vi "GetPosition.vi"(9 "连接ID":refnum<k5>) -> (0 "y":dbl, 1 "x":dbl, 3 "连接ID 2":refnum<k5>, 4 "c":dbl)   [LabVIEW 2016]
panel:
  out "数据输出":string
  in  "错误输入（无错误）":errorcluster
  out "error out":errorcluster
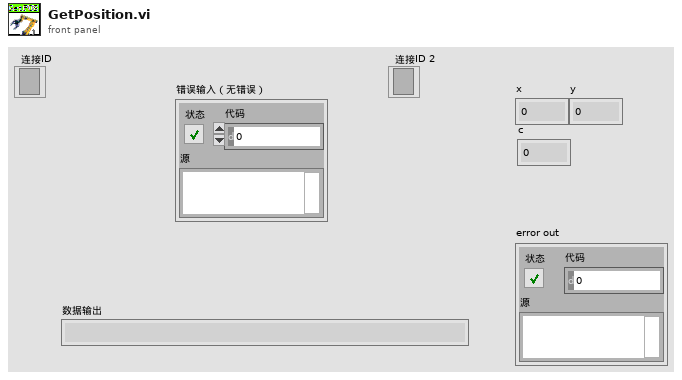
[diagram p1: front panel]
types:
  T1 = enum16{"Standard", "Buffered", "CRLF", "Immediate"}
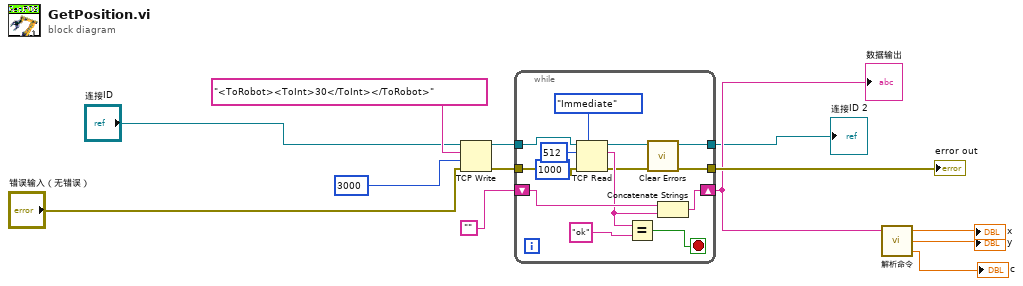
[diagram p0: block diagram]
diagram:
  n1 = TCP Write(connection ID="连接ID", data in="<ToRobot><ToInt>30</ToInt></ToRobot>", error in (no error)="错误输入（无错误）", 9:3000 ("超时毫秒(25000)")) -> (connection ID out=w11:refnum<k5>, error out=w8:errorcluster)  [unwired: 1 out]
  n2 = while {
    shift-right: [w17] -> w7
    shift-left: "" -> [w18]
    tunnel: w11 -> [w25]
    tunnel: [w26] -> w2
    tunnel: w8 -> [w22]
    tunnel: [w15] -> w12
    stop <- w19 stop-if-true
    n3 = TCP Read(connection ID=w25, bytes to read=512 ("读取的字节"), error in (no error)=w22, 7:T1."Immediate" ("模式（标准）"), 9:1000 ("超时毫秒(25000)")) -> (connection ID out=w26:refnum<k5>, data out=w16:string, error out=w14:errorcluster)
    n4 = Equal?(x=w16, y="ok") -> (x = y?=w19:bool)
    n5 = call <vilib>:"Clear Errors.vi"("error in (no error)"=w14) -> ("error out"=w15:errorcluster)  [unwired: 5 in, 1 out]
    n6 = Concatenate Strings(w18, w16) -> (w17:string)
  }
  "error out" <- w12
  "数据输出" <- w7
  "连接ID 2" <- w2
  n7 = call "解析命令.vi"("Robot Status 2"=w7) -> ("C"=→"c":dbl, "y"=→"y":dbl, "x"=→"x":dbl)  [unwired: 2 in]
